vi "Teleop.vi"(10 "Match Info":T1={"Autonomous Elapsed Seconds"=0.0, "TeleOp Elapsed Seconds"=0.0, "Disabled Elapsed Seconds"=0.0, "Visited Autonomous"=FALSE, "Visited TeleOp"=FALSE, "Visited Disabled"=FALSE, "Autonomous Settings"={"Autonomous Style"=enum."Independent", "VI Refnum"=refnum}}, 11 "Call Context":T2) -> ()   [LabVIEW 2020]
doc: "This VI is called for each enabled TeleOp packet received from the DS. It is typically used to read from joysticks and other inputs and update I/O or setpoints for timed control loops. It should complete and return within 20 milliseconds or risk missing DS packets."
uses:
  <vilib>/Rock Robotics/WPI/DriverStation/WPI_DriverStationDerivedRobotMode.ctl
  <vilib>/Rock Robotics/WPI/DriverStation/WPI_DriverStationMatch Info.ctl
  <vilib>/Rock Robotics/WPI/Utilities/WPI_GetSetVariantRefNum.vi
  <vilib>/Rock Robotics/Network Tables/NT Write Boolean Array.vi
  <vilib>/Rock Robotics/Network Tables/NT Write Numeric Array.vi
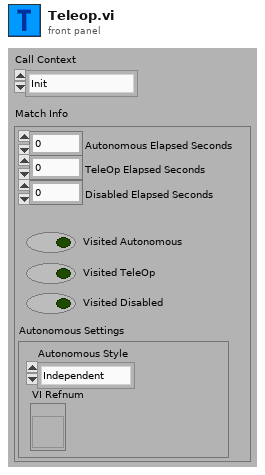
[diagram p1: front panel]
types:
  T1 = typedef "WPI_DriverStationMatch Info.ctl" = cluster{"Autonomous Elapsed Seconds":dbl, "TeleOp Elapsed Seconds":dbl, "Disabled Elapsed Seconds":dbl, "Visited Autonomous":bool, "Visited TeleOp":bool, "Visited Disabled":bool, "Autonomous Settings":cluster{"Autonomous Style":enum16{"Iterative", "Independent"}, "VI Refnum":refnum<vi>}}
  T2 = typedef "WPI_DriverStationDerivedRobotMode.ctl" = enum16{"Init", "Execute", "Stop"}
  T3 = typedef "WPI_JoystickDevRef.ctl" = cluster{"Device":T4}
  T4 = typedef "WPI_JoystickDeviceEnum.ctl" = enum16{"USB 0", "USB 1", "USB 2", "USB 3", "USB 4", "USB 5"}
  T5 = typedef "Command Status Info.ctl" = cluster{"Name":string, "Status":T6, "notifier out":T7}
  T6 = typedef "Completion Status.ctl" = enum16{"Successful", "Aborted", "Incomplete"}
  T7 = typedef "Completion Notifier.ctl" = refnum<notifier>
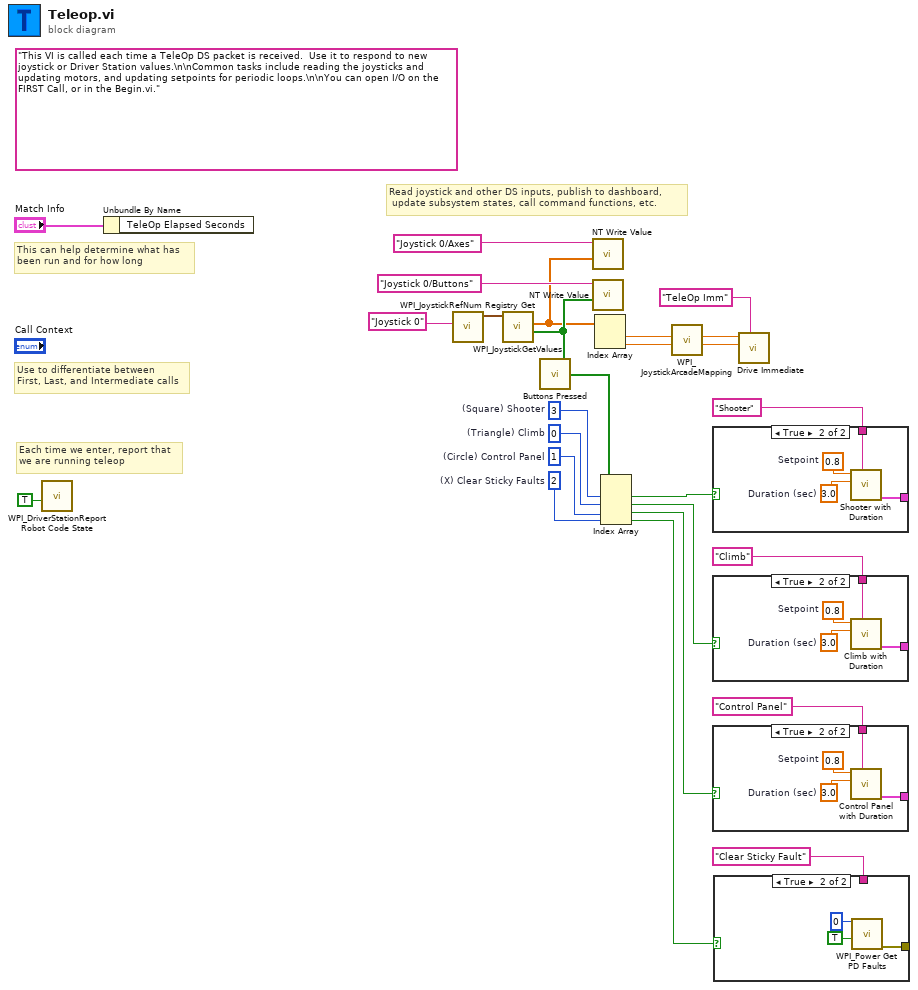
[diagram p0: block diagram]
diagram:
  w4 = 2  # (X) Clear Sticky Faults
  w5 = 1  # (Circle) Control Panel
  w6 = 0  # (Triangle) Climb
  w7 = 3  # (Square) Shooter
  (unwired) "This VI is called each time a TeleOp DS packet is received.  Use it to respond to new joystick or Driver Station values.\n\nCommon tasks include reading the joysticks and updating motors, and updating setpoints for periodic loops.\n\nYou can open I/O on the FIRST Call, or in the Begin.vi."
  # "Read joystick and other DS inputs, publish to dashboard,\n update subsystem states, call command functions, etc."
  # "Each time we enter, report that\nwe are running teleop"
  # "Use to differentiate between\nFirst, Last, and Intermediate calls"
  # "This can help determine what has\nbeen run and for how long"
  n1 = call <vilib>:"WPI_DriverStationReport Robot Code State.vi"("TeleOp"=TRUE ("Autonomous")) -> ()  [unwired: 10 in, 1 out]
  n2 = Unbundle By Name("Match Info") -> ()  [unwired: 1 out]
  n3 = call <vilib>:"WPI_JoystickRefNum Registry Get.vi"("refnum name"="Joystick 0") -> ("JoystickDevRef"=w23:T3)  [unwired: 1 in, 9 out]
  n4 = call <vilib>:"WPI_JoystickGetValues.vi"("JoystickDevRef"=w23) -> ("Buttons"=w13:bool[], "Axes"=w12:dbl[])  [unwired: 6 in, 3 out]
  n5 = call "Buttons Pressed.vi"("Button Values"=w13) -> ("Button Presses"=w20:bool[])
  n6 = call-poly <vilib>:"NT Write Value.vi"("Numeric Array"=w12, "Name"="Joystick 0/Axes") -> ()  [unwired: 9 in, 1 out]
  n7 = call-poly <vilib>:"NT Write Value.vi"("Boolean Array"=w13, "Name"="Joystick 0/Buttons") -> ()  [unwired: 9 in, 1 out]
  n8 = Index Array(array=w12) -> (element #1=w16:dbl, element #2=w15:dbl)  [unwired: 2 in]
  n9 = Index Array(array=w20, index #1=w7, index #2=w6, index #3=w5, index #4=w4) -> (element #1=w19:bool, element #2=w3:bool, element #3=w2:bool, element #4=w1:bool)
  n10 = call <vilib>:"WPI_JoystickArcadeMapping.vi"("Y axis value"=w15, "X axis value"=w16) -> ("Right Motor Value"=w17:dbl, "Left Motor Value"=w18:dbl)  [unwired: 8 in]
  n11 = case shown="True" w19 {
    tunnel: [_ w30] -> _
    tunnel: "Shooter" ("Description") -> [_ w29]
    frame False {
    }
    frame True {
      w27 = 3.0  # Duration (sec)
      w28 = 0.8  # Setpoint
      n12 = call "Shooter with Duration.vi"("Description"=w29, "Duration (s)"=w27, "Setpoint"=w28) -> ("Command Info Out"=w30:T5)  [unwired: 8 in]
    }
  }
  n13 = case shown="True" w3 {
    tunnel: [_ w34] -> _
    tunnel: "Climb" ("Description") -> [_ w33]
    frame False {
    }
    frame True {
      w31 = 3.0  # Duration (sec)
      w32 = 0.8  # Setpoint
      n14 = call "Climb with Duration.vi"("Description"=w33, "Duration (s)"=w31, "Setpoint"=w32) -> ("Command Info Out"=w34:T5)  [unwired: 8 in]
    }
  }
  n15 = case shown="True" w2 {
    tunnel: [_ w38] -> _
    tunnel: "Control Panel" ("Description") -> [_ w37]
    frame False {
    }
    frame True {
      w35 = 3.0  # Duration (sec)
      w36 = 0.8  # Setpoint
      n16 = call "Control Panel with Duration.vi"("Description"=w37, "Duration (s)"=w35, "Setpoint"=w36) -> ("Command Info Out"=w38:T5)  [unwired: 8 in]
    }
  }
  n17 = case shown="True" w1 {
    tunnel: [_ w41] -> _
    tunnel: "Clear Sticky Fault" ("Description") -> [_ _]
    frame False {
    }
    frame True {
      n18 = call <vilib>:"WPI_Power Get PD Faults.vi"("Power Distribution (def)"=u8 0, "Clear Sticky Faults"=TRUE) -> ("error out"=w41:errorcluster)  [unwired: 10 in, 3 out]
    }
  }
  n19 = call "Drive Immediate.vi"("Description"="TeleOp Imm", "Right Setpoint"=w17, "Left Setpoint"=w18) -> ()  [unwired: 8 in, 1 out]
